vi "Test_PublicationLocked_PublisherOwnsLock_OK.vi"(8 "error in (no error)":errorcluster, 11 "TestMediator In":refnum<class "TestMediator.lvclass">) -> (0 "error out":errorcluster, 3 "TestMediator Out":refnum<class "TestMediator.lvclass">)   [LabVIEW 2015, in "TestMediator.lvclass"]
uses:
  TestMediator.lvclass
  Mediator/Mediator.lvclass
  IMediator/PublishRequest/PublishRequest.lvclass/PublishRequest.ctl
  Transport/QueueTransport/QueueTransport.lvclass/QueueTransport.ctl
  SubscriptionPolicy/BasicSubscription/BasicSubscription.lvclass/BasicSubscription.ctl
  IMediator/SubscriptionRequest/SubscriptionRequest.lvclass/SubscriptionRequest.ctl
  IMediator/IMediator Messages/Lock Publication Msg/Lock Publication Msg.lvclass/Lock Publication Msg.ctl
  <vilib>/ActorFramework/Message Enqueuer/Message Enqueuer.lvclass/Message Enqueuer.ctl
  IMediator/IMediator Messages/Publish Msg/Publish Msg.lvclass/Publish Msg.ctl
  IMediator/IMediator Messages/Subscribe Msg/Subscribe Msg.lvclass/Subscribe Msg.ctl
  <vilib>/ActorFramework/Message Enqueuer/Enqueue.vi
  <vilib>/Utility/error.llb/Error Cluster From Error Code.vi
  <vilib>/ActorFramework/Message Priority Queue/Priority Enqueue.vi
  SubscriptionPolicy/BasicSubscription/BasicSubscription.lvclass
  Transport/QueueTransport/QueueTransport.lvclass
  IMediator/SubscriptionRequest/SubscriptionRequest.lvclass
  IMediator/IPublicationPolicy/IPublicationPolicy.lvclass
  IMediator/ITransport/ITransport.lvclass
  IMediator/IMediator Messages/Lock Publication Msg/Lock Publication Msg.lvclass
  IMediator/PublishRequest/PublishRequest.lvclass
  IMediator/IMediator Messages/Publish Msg/Publish Msg.lvclass
  IMediator/IMediator Messages/Subscribe Msg/Subscribe Msg.lvclass
  <vilib>/ActorFramework/Stop Msg/Stop Msg.lvclass
  <vilib>/addons/_JKI Toolkits/VI Tester/TestCase.llb/TestCase.lvclass
  <vilib>/ActorFramework/Actor/Actor.lvclass
  IMediator/ISubscriptionPolicy/ISubscriptionPolicy.lvclass
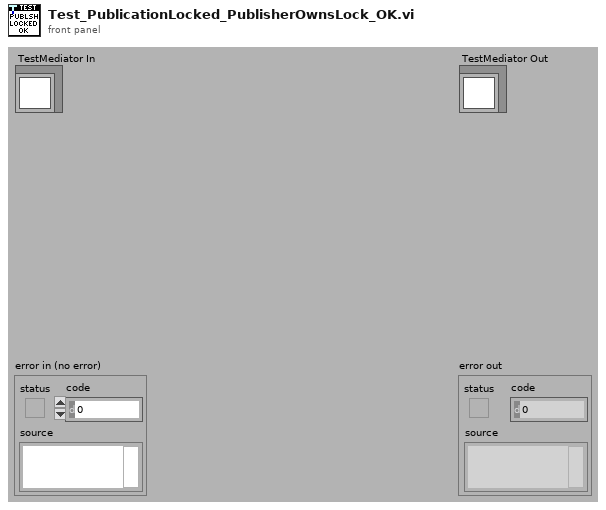
[diagram p1: front panel]
types:
  T1 = typedef "IMediator.lvlib/ISubscriptionPolicy.lvclass/ISubscriptionPolicy Reference.ctl" = refnum<data-value>
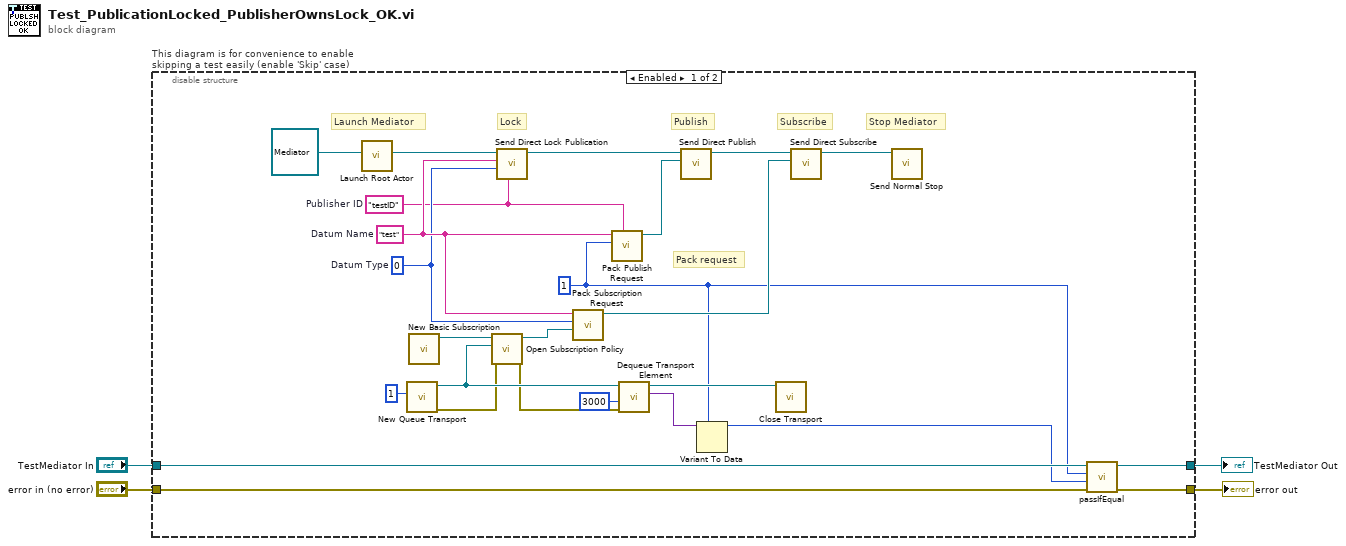
[diagram p0: block diagram]
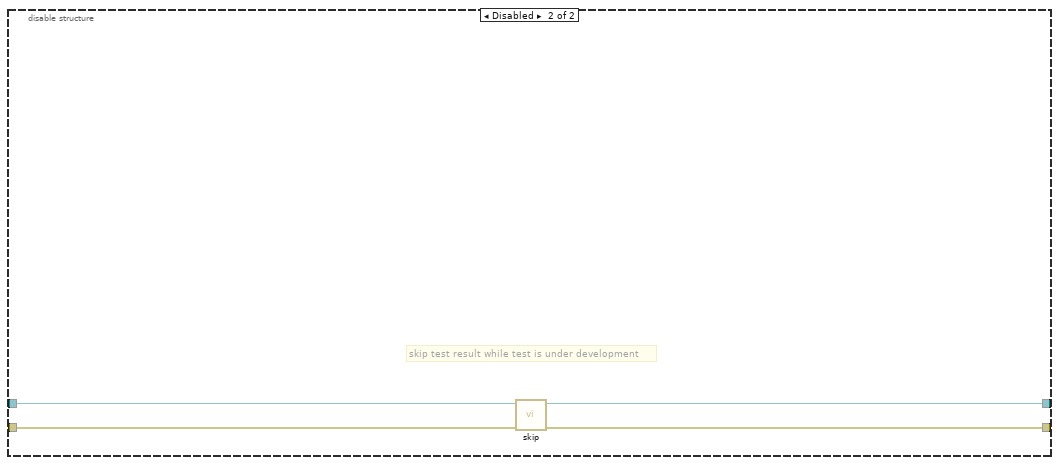
[diagram p2: hidden frame]
diagram:
  n1 = disable-structure "This diagram is for convenience to enable skipping a test easily (enable 'Skip' case)" shown="Enabled" {
    disable-tunnel: "TestMediator In" -> [w29 w33]
    disable-tunnel: [w28 w31] -> w1
    disable-tunnel: [w27 w32] -> w3
    disable-tunnel: "error in (no error)" -> [w26 w30]
    frame Enabled {
      w5 = "testID"  # Publisher ID
      w6 = 0  # Datum Type
      w7 = "test"  # Datum Name
      w10 = 1
      # "Pack request"
      # "Lock"
      # "Launch Mediator"
      # "Stop Mediator"
      # "Subscribe"
      # "Publish"
      n2 = call <vilib>:"Launch Root Actor.vi"("Actor"=refnum<class "Mediator.lvclass"> refnum ("Mediator.lvlib:Mediator.lvclass")) -> ("Actor's Enqueuer"=w24:refnum<class "Message Enqueuer.lvclass">)  [unwired: 9 in, 1 out]
      n3 = call "New Queue Transport.vi"("Max Queue Size (-1)"=1) -> ("error out"=w18:errorcluster, "QueueTransport"=w20:refnum<class "QueueTransport.lvclass">)  [unwired: 9 in]
      n4 = call "New Basic Subscription.vi"() -> ("BasicSubscription Out"=w12:refnum<class "BasicSubscription.lvclass">)  [unwired: 11 in]
      n5 = call "Open Subscription Policy.vi"("error in (no error)"=w18, "Transport"=w20, "SubscriptionPolicy"=w12) -> ("error out"=w17:errorcluster, "Subscription Policy"=w11:T1)  [unwired: 7 in]
      n6 = call "Send Direct Lock Publication.vi"("Publisher ID"=w5, "Datum Type"=w6, "Datum Name"=w7, "Mediator Enqeuer"=w24) -> ("Mediator Enqueuer out"=w8:refnum<class "Message Enqueuer.lvclass">)  [unwired: 6 in, 1 out]
      n7 = call "Pack Subscription Request.vi"("Subscription Policy"=w11, "Type"=w6, "Datum Name"=w7) -> ("SubscriptionRequest"=w23:refnum<class "SubscriptionRequest.lvclass">)  [unwired: 8 in]
      n8 = call "Pack Publish Request.vi"("Publisher ID"=w5, "Data to Publish"=w10, "Datum Name"=w7) -> ("PublishRequest"=w9:refnum<class "PublishRequest.lvclass">)  [unwired: 8 in]
      n9 = call "Dequeue Transport Element.vi"("error in (no error)"=w17, "Timeout In ms (-1)"=3000, "QueueTransport in"=w20) -> ("Data"=w14:variant, "QueueTransport out"=w15:refnum<class "QueueTransport.lvclass">)  [unwired: 5 in, 2 out]
      n10 = call "Send Direct Publish.vi"("PublishRequest"=w9, "Mediator Enqeuer"=w8) -> ("Mediator Enqueuer out"=w22:refnum<class "Message Enqueuer.lvclass">)  [unwired: 8 in, 1 out]
      n11 = Variant To Data(type=w10, Variant=w14) -> (data=w13:i32)  [unwired: 1 in, 1 out]
      n12 = call-dynamic "Close Transport.vi"("QueueTransport in"=w15) -> ()  [unwired: 10 in, 1 out]
      n13 = call "Send Direct Subscribe.vi"("Subscription Request"=w23, "Message Enqueuer"=w22) -> ("Message Enqueuer out"=w16:refnum<class "Message Enqueuer.lvclass">)  [unwired: 8 in, 1 out]
      n14 = call <vilib>:"Send Normal Stop.vi"("Message Enqueuer"=w16) -> ()  [unwired: 10 in, 1 out]
      n15 = call-dynamic "passIfEqual.vi"("error in (no error)"=w26, "y"=w13, "x"=w10, "TestCase in"=w29) -> ("error out"=w27:errorcluster, "TestCase out"=w28:refnum<class "TestMediator.lvclass">)  [unwired: 6 in]
    }
    frame Disabled {
      # "skip test result while test is under development"
      n16 = call <vilib>:"skip.vi"("error in (no error)"=w30, "TestCase in"=w33) -> ("error out"=w32:errorcluster, "TestCase out"=w31:refnum<class "TestMediator.lvclass">)  [unwired: 8 in]
    }
  }
  "error out" <- w3
  "TestMediator Out" <- w1
